vi "Test-aesb_single_round.vi"() -> ()   [LabVIEW 2017]
panel:
  out "exp_c":u32[](array[numeric]) format="%.0x"
  out "exp_a":u32[](array[numeric]) format="%.0x"
  out "_c":u32[](array[numeric]) format="%.0x"
  out "_a":u32[](array[numeric]) format="%.0x"
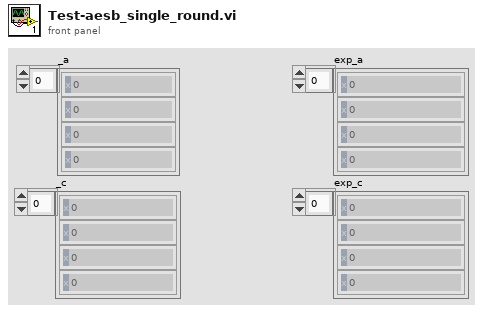
[diagram p1: front panel]
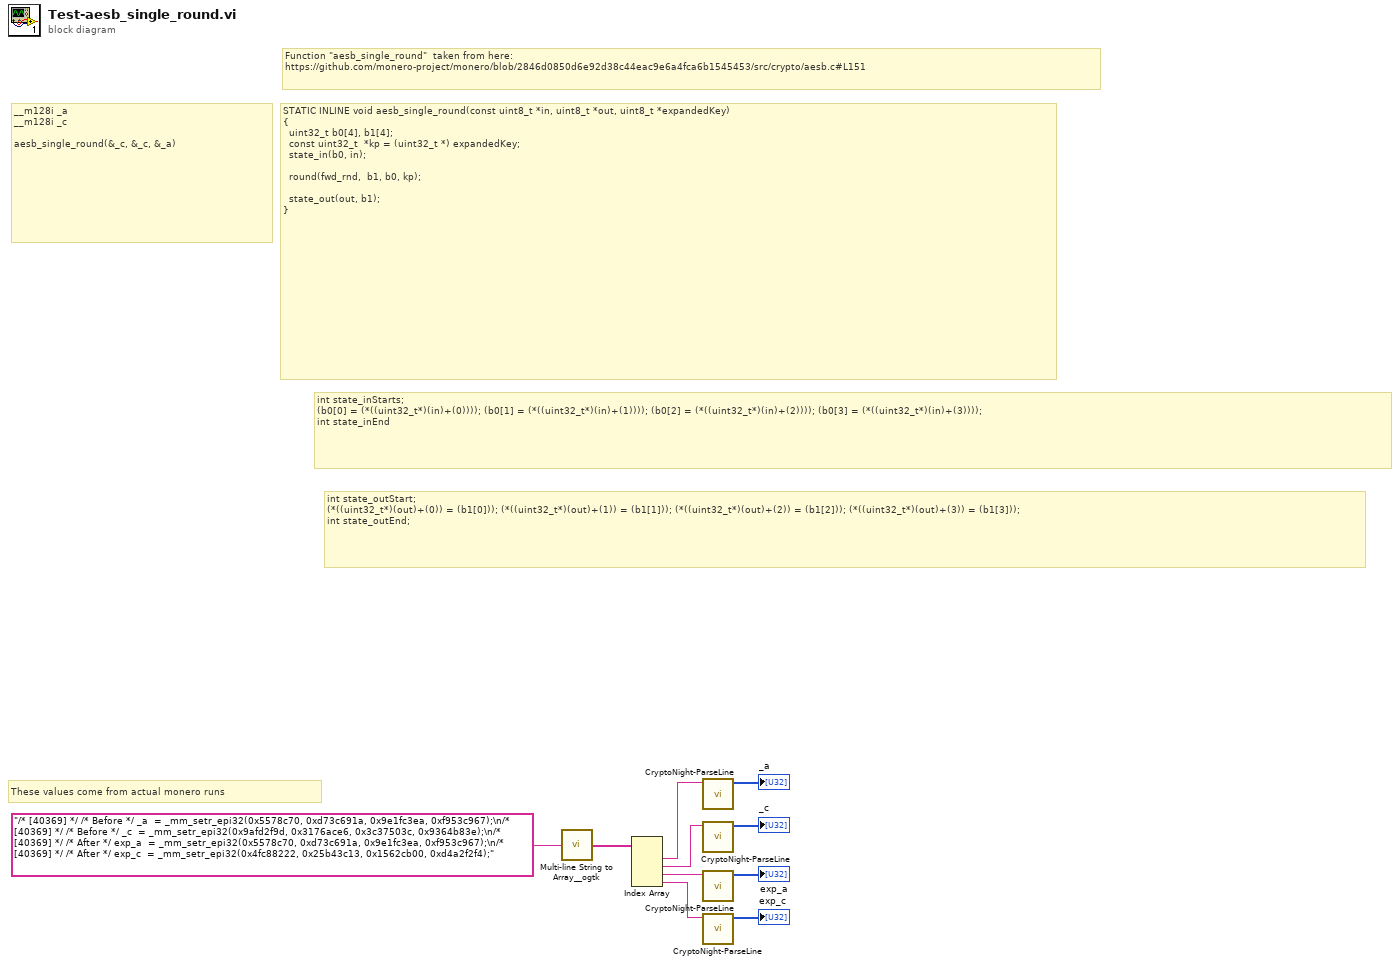
[diagram p0: block diagram]
diagram:
  # "These values come from actual monero runs"
  # "int state_outStart;\n(*((uint32_t*)(out)+(0)) = (b1[0])); (*((uint32_t*)(out)+(1)) = (b1[1])); (*((uint32_t*)(out)+(2)) = (b1[2])); (*((uint32_t*)(out)+(3)) = (b1[3]));\nint state_outEnd;"
  # "int state_inStarts;\n(b0[0] = (*((uint32_t*)(in)+(0)))); (b0[1] = (*((uint32_t*)(in)+(1)))); (b0[2] = (*((uint32_t*)(in)+(2)))); (b0[3] = (*((uint32_t*)(in)+(3))));\nint state_inEnd"
  # "Function \"aesb_single_round\"  taken from here:\nhttps://github.com/monero-project/monero/blob/2846d0850d6e92d38c44eac9e6a4fca6b1545453/src/crypto/aesb.c#L151"
  # "STATIC INLINE void aesb_single_round(const uint8_t *in, uint8_t *out, uint8_t *expandedKey)\n{\n  uint32_t b0[4], b1[4];\n  const uint32_t  *kp = (uint32_t *) expandedKey;\n  state_in(b0, in);\n\n  round(fwd_rnd,  b1, b0, kp);\n\n  state_out(out, b1);\n}"
  # "__m128i _a\n__m128i _c\n\naesb_single_round(&_c, &_c, &_a)"
  n1 = call <userlib>:"Multi-line String to Array__ogtk.vi"("string"="/* [40369] */ /* Before */ _a  = _mm_setr_epi32(0x5578c70, 0xd73c691a, 0x9e1fc3ea, 0xf953c967);\n/* [40369] */ /* Before */ _c  = _mm_setr_epi32(0x9afd2f9d, 0x3176ace6, 0x3c37503c, 0x9364b83e);\n/* [40369] */ /* After */ exp_a  = _mm_setr_epi32(0x5578c70, 0xd73c691a, 0x9e1fc3ea, 0xf953c967);\n/* [40369] */ /* After */ exp_c  = _mm_setr_epi32(0x4fc88222, 0x25b43c13, 0x1562cb00, 0xd4a2f2f4);") -> ("lines"=w1:string[])
  n2 = Index Array(array=w1) -> (element #1=w10:string, element #2=w8:string, element #3=w7:string, element #4=w6:string)  [unwired: 4 in]
  n3 = call "CryptoNight-ParseLine.vi"("line"=w10) -> ("Array"=→"_a":u32[])  [unwired: 10 in]
  n4 = call "CryptoNight-ParseLine.vi"("line"=w8) -> ("Array"=→"_c":u32[])  [unwired: 10 in]
  n5 = call "CryptoNight-ParseLine.vi"("line"=w7) -> ("Array"=→"exp_a":u32[])  [unwired: 10 in]
  n6 = call "CryptoNight-ParseLine.vi"("line"=w6) -> ("Array"=→"exp_c":u32[])  [unwired: 10 in]
